vi "invertInput_8bit.vi"(0 "R2":bool, 1 "R3":bool, 2 "R4":bool, 3 "R5":bool, 4 "R6":bool, 5 "R7":bool, 6 "R1":bool, 7 "R8":bool) -> (12 "R7":bool, 13 "R8":bool, 14 "R1":bool, 15 "R2":bool, 16 "R3":bool, 17 "R4":bool, 18 "R5":bool, 19 "R6":bool)   [LabVIEW 2019]
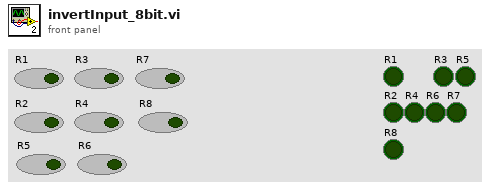
[diagram p1: front panel]
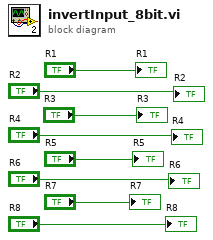
[diagram p0: block diagram]
diagram:
  "R1" <- "R1"
  "R2" <- "R2"
  "R3" <- "R3"
  "R4" <- "R4"
  "R5" <- "R5"
  "R6" <- "R6"
  "R7" <- "R7"
  "R8" <- "R8"
